vi "ParseArguments.vi"(8 "error in (no error)":errorcluster, 10 "Inputs":string[](array[string]), 11 "RunUnitTests in":refnum<class "RunUnitTests.lvclass">) -> (0 "error out":errorcluster, 3 "RunUnitTests out":refnum<class "RunUnitTests.lvclass">)   [LabVIEW 2014, in "RunUnitTests.lvclass"]
uses:
  RunUnitTests.lvclass
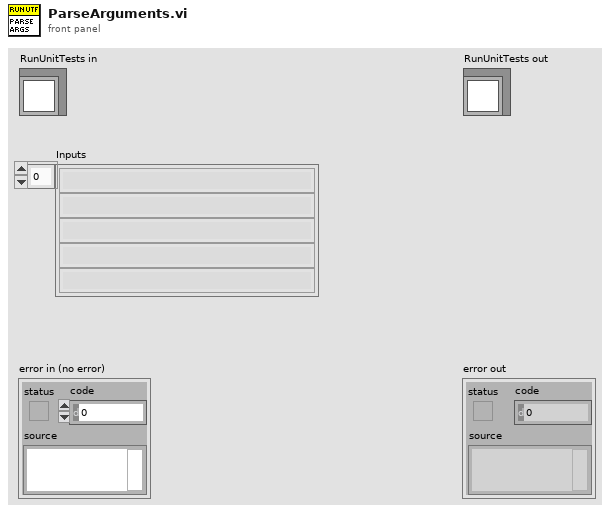
[diagram p1: front panel]
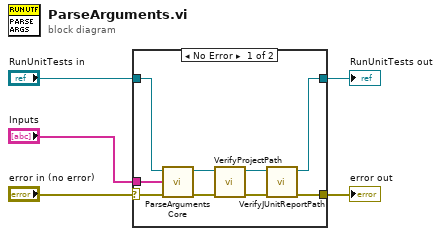
[diagram p0: block diagram]
diagram:
  n1 = case shown="No Error" "error in (no error)" {
    selector: "error in (no error)" -> [w12 w16]
    tunnel: [w6 w16] -> w4
    tunnel: "RunUnitTests in" -> [w13 w15]
    tunnel: [w8 w15] -> w1
    tunnel: "Inputs" -> [w14 _]
    frame No Error {
      n2 = call "ParseArgumentsCore.vi"("error in (no error)"=w12, "Inputs"=w14, "RunUnitTests in"=w13) -> ("error out"=w11:errorcluster, "RunUnitTests out"=w10:refnum<class "RunUnitTests.lvclass">)  [unwired: 7 in]
      n3 = call "VerifyProjectPath.vi"("error in (no error)"=w11, "RunUnitTests in"=w10) -> ("error out"=w9:errorcluster, "RunUnitTests out"=w7:refnum<class "RunUnitTests.lvclass">)  [unwired: 8 in]
      n4 = call "VerifyJUnitReportPath.vi"("error in (no error)"=w9, "RunUnitTests in"=w7) -> ("error out"=w6:errorcluster, "RunUnitTests out"=w8:refnum<class "RunUnitTests.lvclass">)  [unwired: 8 in]
    }
    frame Error {
    }
  }
  "error out" <- w4
  "RunUnitTests out" <- w1
